vi "Open Demosaicker.vi"(8 "error in (no error)":errorcluster) -> (0 "error out":errorcluster, 3 "Demosaicker reference":refnum<k24>)   [LabVIEW 2015]
uses:
  C:/code/Host/Installer/Scientific Camera Interfaces/LabVIEW/32_bit/Library_X86/Thorlabs.TSI.Demosaicker.dll
  32_bit/Library_X86/Thorlabs.TSI.Demosaicker.dll
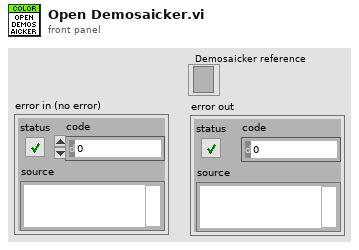
[diagram p1: front panel]
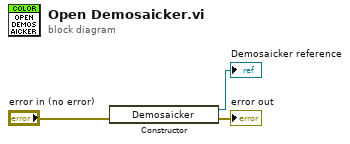
[diagram p0: block diagram]
diagram:
  n1 = constructor class="Demosaicker"(error in="error in (no error)") -> (reference out=→"Demosaicker reference":refnum<k24>, error out=→"error out":errorcluster)  [unwired: 2 in, 1 out]
